vi "Subject2Path.vi"(0 "Subject Initials":string) -> (2 "Subject Root":path, 3 "Data Path":path, 4 "Calibration Path":path)   [LabVIEW 2012]
doc: "Loads the Root path of the data from global variables and returns subject specific data paths to contain the data and calibration measurements."
uses:
  GlobalVariables.vi
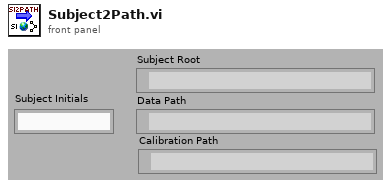
[diagram p1: front panel]
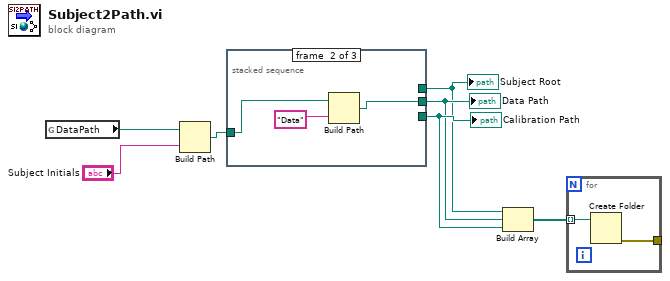
[diagram p0: block diagram]
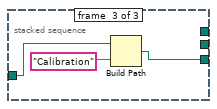
[diagram p3: hidden frame]
diagram:
  n1 = global read "GlobalVariables.vi" "DataPath"() -> (w7:path)
  n2 = Build Path(base path=w7, name or relative path="Subject Initials") -> (appended path=w5:path)
  n3 = stacked-sequence {
    tunnel: w5 -> [w8 w11 w14]
    tunnel: [w8 _ _] -> w2
    tunnel: [_ w9 _] -> w3
    tunnel: [_ _ w12] -> w4
    frame #0 {
    }
    frame #1 {
      n4 = Build Path(base path=w11, name or relative path="Data") -> (appended path=w9:path)
    }
    frame #2 {
      n5 = Build Path(base path=w14, name or relative path="Calibration") -> (appended path=w12:path)
    }
  }
  "Subject Root" <- w2
  "Data Path" <- w3
  "Calibration Path" <- w4
  n6 = Build Array(w2, w3, w4) -> (w1:path[])
  n7 = for {
    tunnel: w1 -> [w16] mode=indexing
    tunnel: [w15] -> _
    n8 = Create Folder(path (use dialog)=w16) -> (error out=w15:errorcluster)  [unwired: 2 in, 2 out]
  }
